vi "SRV_Start Sensors_Build Sensors Commands Arrays.vi"(0 "Sensors Config":T3[](array[typedef]) {"Register" format="%.0x"; "I2C Address" format="%.0x"; "Sample Period (ms)" min=10 max=60000 step=1; "Digital Mask" format="%.0x"; "Channel" format="%.0x"}, 11 "error in (no error)":errorcluster) -> (2 "Streaming Sensor View Indicator Names":T1[](array[typedef]), 3 "Polled Sensor View Indicator Names":T1[](array[typedef]), 6 "Active Streaming Cfg-Commands":T2[](array[typedef]) {"Calculated Sensors Array"."Parsed Formula"."Y Values" format="%.2f"; "Calculated Sensors Array"."Sensor Config"."Register" format="%.0x"; "Calculated Sensors Array"."Sensor Config"."I2C Address" format="%.0x"; "Calculated Sensors Array"."Sensor Config"."Sample Period (ms)" min=10 max=60000 step=1; "Calculated Sensors Array"."Sensor Config"."Digital Mask" format="%.0x"; "Calculated Sensors Array"."Sensor Config"."Channel" format="%.0x"; "Parsed Formula"."Y Values" format="%.2f"; "Sensor Config"."Register" format="%.0x"; "Sensor Config"."I2C Address" format="%.0x"; "Sensor Config"."Sample Period (ms)" min=10 max=60000 step=1; "Sensor Config"."Digital Mask" format="%.0x"; "Sensor Config"."Channel" format="%.0x"}, 10 "Active Polled Cfg-Commands":T2[](array[typedef]) {"Calculated Sensors Array"."Parsed Formula"."Y Values" format="%.2f"; "Calculated Sensors Array"."Sensor Config"."Register" format="%.0x"; "Calculated Sensors Array"."Sensor Config"."I2C Address" format="%.0x"; "Calculated Sensors Array"."Sensor Config"."Sample Period (ms)" min=10 max=60000 step=1; "Calculated Sensors Array"."Sensor Config"."Digital Mask" format="%.0x"; "Calculated Sensors Array"."Sensor Config"."Channel" format="%.0x"; "Parsed Formula"."Y Values" format="%.2f"; "Sensor Config"."Register" format="%.0x"; "Sensor Config"."I2C Address" format="%.0x"; "Sensor Config"."Sample Period (ms)" min=10 max=60000 step=1; "Sensor Config"."Digital Mask" format="%.0x"; "Sensor Config"."Channel" format="%.0x"}, 15 "error out":errorcluster)   [LabVIEW 2009]
uses:
  SRV_Sensor Config Cluster.ctl
  SRV_Sensor Analog-Digital.ctl
  SRV_Sensor Sampling Mode.ctl
  SRV_Sensor View Config Cluster.ctl
  SRV_Sensors Names.ctl
  SRV_Sensor PicoC Shared Var Type.ctl
  SRV_Sensor Number of Bytes.ctl
  SRV_Sensor Integer Word Type.ctl
  SRV_Sensor Config-Command Cluster.ctl
  SRV_Calculated Sensor Cfg.ctl
panel:
  # "operator"
  # "register1"
  # "register2"
  # "operator"
  # "register1"
  # "register2"
  # "operator"
  # "register1"
  # "register2"
  # "operator"
  # "register1"
  # "register2"
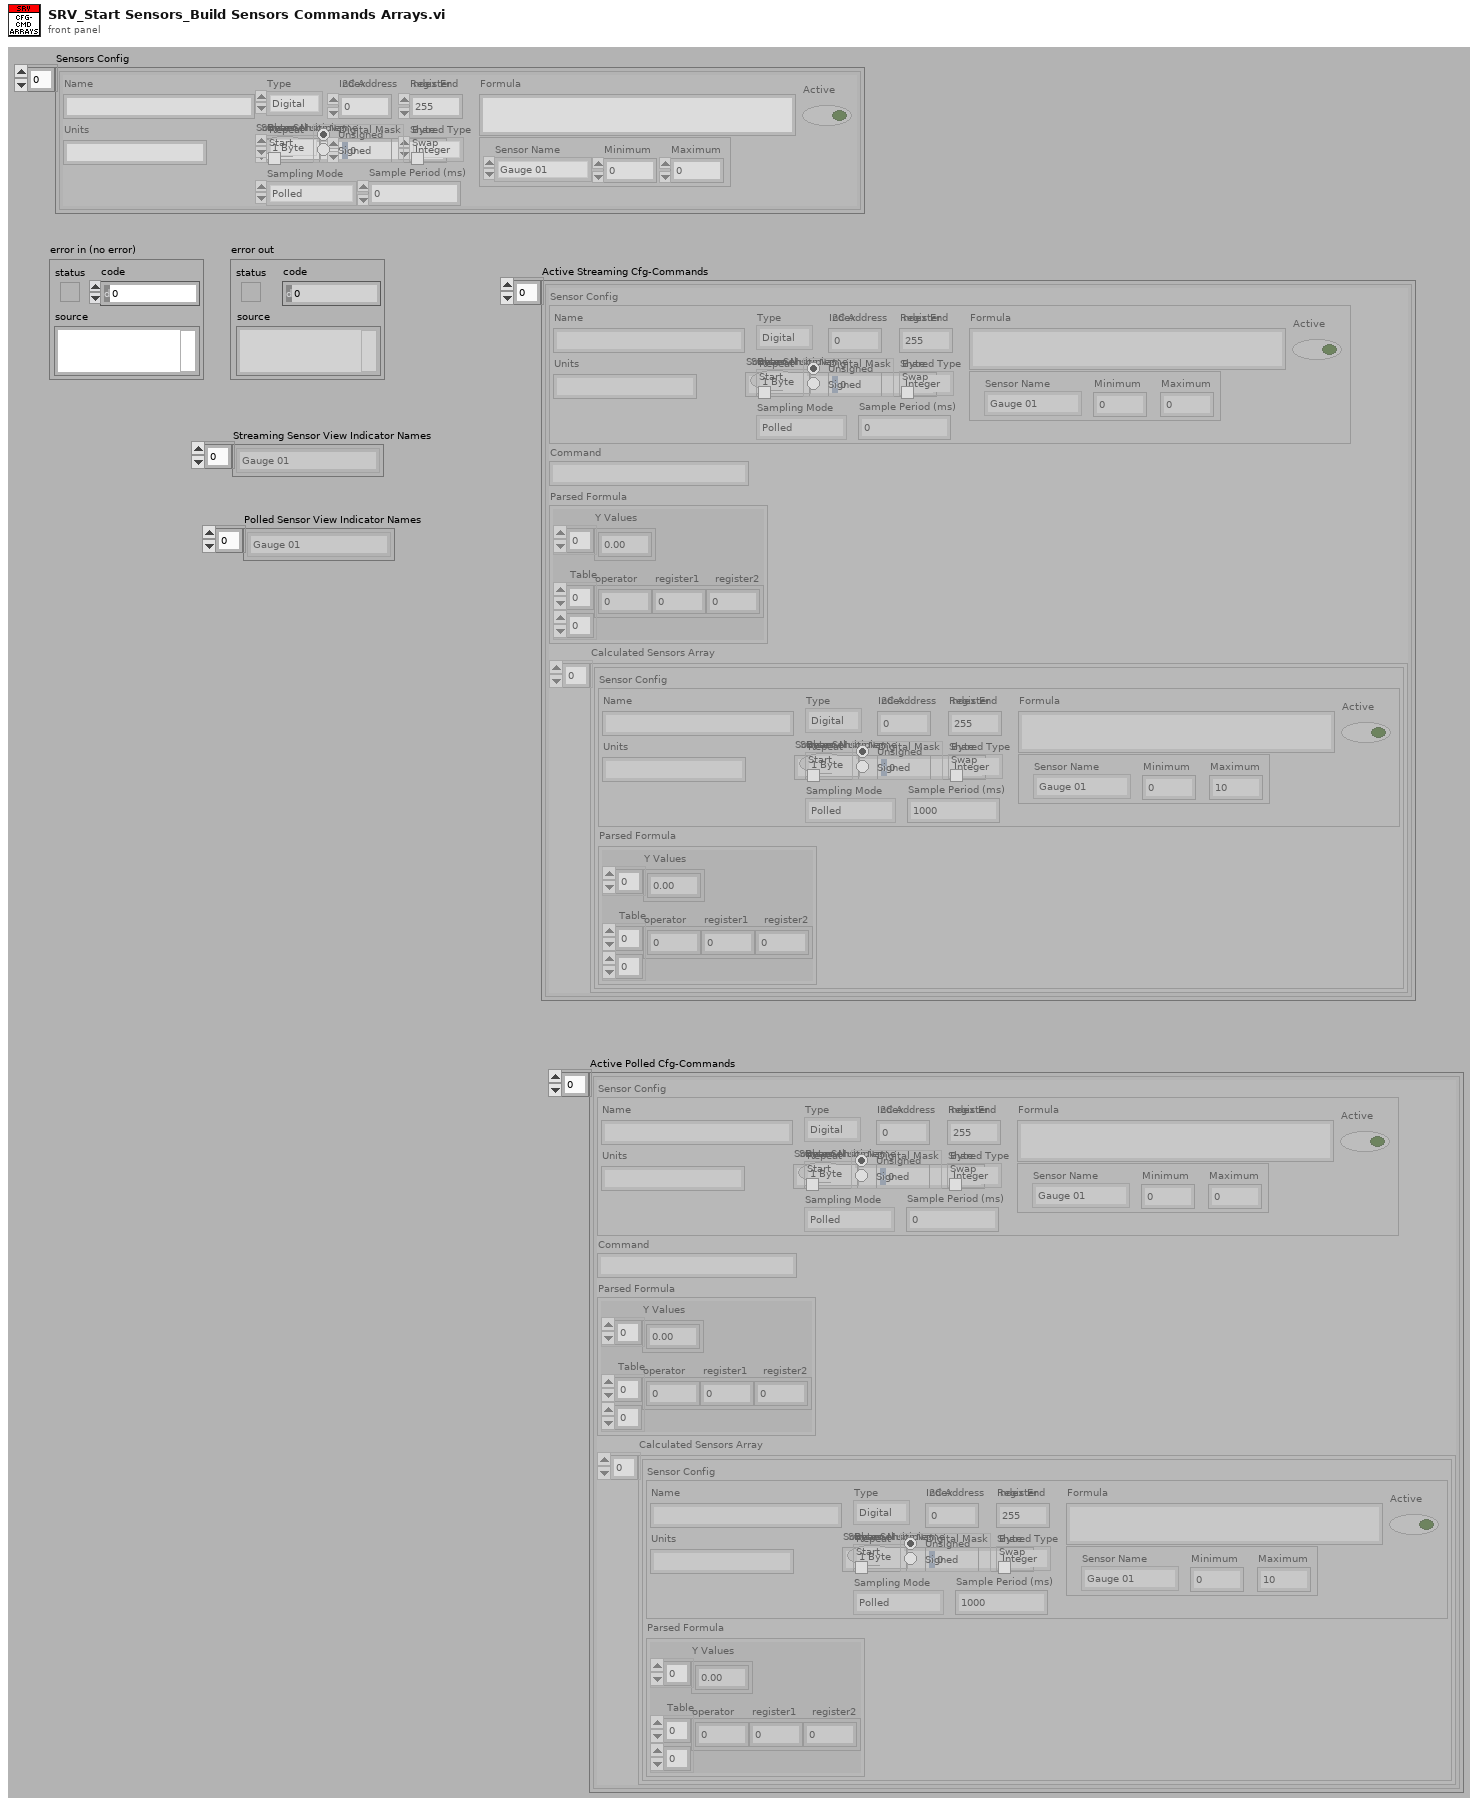
[diagram p1: front panel]
types:
  T1 = typedef "SRV_Sensors Names.ctl" = enum16{"Gauge 01", "Gauge 02", "Gauge 03", "Gauge 04", "Meter 01", "Meter 02", "Meter 03", "Meter 04", "Numeric 01", "Numeric 02", "Numeric 03", "Numeric 04", "Numeric 05", "Numeric 06", "Numeric 07", "Numeric 08", "Boolean 01", "Boolean 02", "Boolean 03", "Boolean 04", "Boolean 05", "Boolean 06", "Boolean 07", "Boolean 08", "Boolean 09", "Boolean 10", "Boolean 11", "Boolean 12", "Boolean 13", "Boolean 14", "Boolean 15", "Boolean 16", "Boolean 17", "Boolean 18", "Boolean 19", "Boolean 20", "Boolean 21", "Boolean 22", "Boolean 23", "Boolean 24", "Boolean 25", "Boolean 26", "Boolean 27", "Boolean 28", "Boolean 29", "Boolean 30", "Boolean 31", "Boolean 32"}
  T2 = typedef "SRV_Sensor Config-Command Cluster.ctl" = cluster{"Sensor Config":T3, "Command":string, "Parsed Formula":cluster{"Table":i32[][], "Y Values":dbl[]}, "Calculated Sensors Array":T10[]}
  T3 = typedef "SRV_Sensor Config Cluster.ctl" = cluster{"Name":string, "A/D":T4, "I2C Address":u8, "Register":u8, "Channel":u8, "Digital Mask":u16, "Units":string, "Sampling Mode":T5, "Sample Period (ms)":u32, "Formula":string, "Sensor View Config":T6, "Active":bool, "PicoC Shared Var Type":T7, "Index":u8, "Stream Multiple?":bool, "Index End":u8, "Bytes":T8, "Source Sensor Name":string, "Repeat Start":bool, "Integer Word Type":T9, "Byte Swap":bool}
  T4 = typedef "SRV_Sensor Analog-Digital.ctl" = enum16{"Digital", "Analog", "PicoC Shared", "Calculated"}
  T5 = typedef "SRV_Sensor Sampling Mode.ctl" = enum16{"Polled", "Streaming"}
  T6 = typedef "SRV_Sensor View Config Cluster.ctl" = cluster{"Sensor Name":T1, "Minimum":dbl, "Maximum":dbl}
  T7 = typedef "SRV_Sensor PicoC Shared Var Type.ctl" = enum16{"String", "Integer", "Float"}
  T8 = typedef "SRV_Sensor Number of Bytes.ctl" = enum16{"1 Byte", "2 Bytes"}
  T9 = typedef "SRV_Sensor Integer Word Type.ctl" = enum32{"Unsigned", "Signed"}
  T10 = typedef "SRV_Calculated Sensor Cfg.ctl" = cluster{"Sensor Config":T3, "Parsed Formula":cluster{"Table":i32[][], "Y Values":dbl[]}}
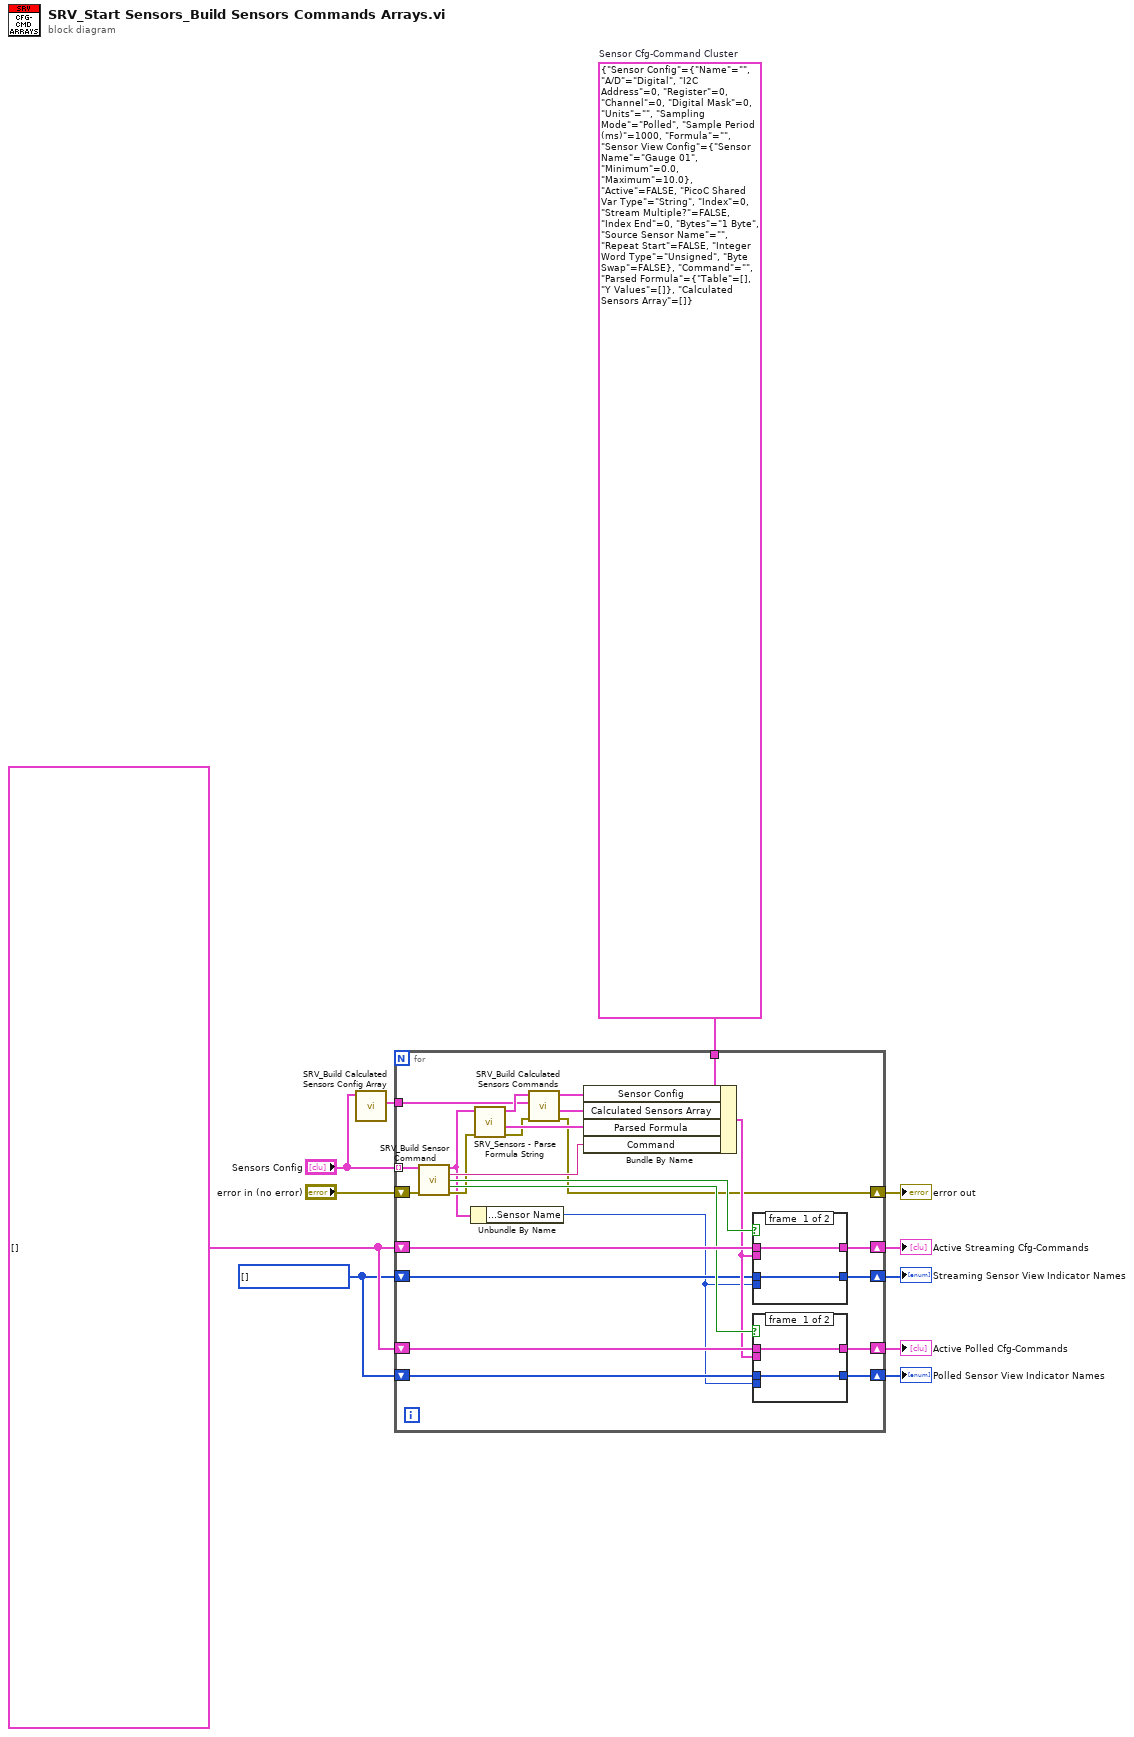
[diagram p0: block diagram]
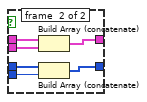
[diagram p2: hidden frame]
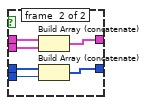
[diagram p3: hidden frame]
diagram:
  w2 = T1[] [] items=["Gauge 01", "Gauge 02", "Gauge 03", "Gauge 04", "Meter 01", "Meter 02", "Meter 03", "Meter 04", "Numeric 01", "Numeric 02", "Numeric 03", "Numeric 04", "Numeric 05", "Numeric 06", "Numeric 07", "Numeric 08", "Boolean 01", "Boolean 02", "Boolean 03", "Boolean 04", "Boolean 05", "Boolean 06", "Boolean 07", "Boolean 08", "Boolean 09", "Boolean 10", "Boolean 11", "Boolean 12", "Boolean 13", "Boolean 14", "Boolean 15", "Boolean 16", "Boolean 17", "Boolean 18", "Boolean 19", "Boolean 20", "Boolean 21", "Boolean 22", "Boolean 23", "Boolean 24", "Boolean 25", "Boolean 26", "Boolean 27", "Boolean 28", "Boolean 29", "Boolean 30", "Boolean 31", "Boolean 32"] ("Sensor View Indicator Names")
  w8 = T2[] []
  w11 = T2 {"Sensor Config"={"Name"="", "A/D"=enum."Digital", "I2C Address"=0, "Register"=0, "Channel"=0, "Digital Mask"=0, "Units"="", "Sampling Mode"=enum."Polled", "Sample Period (ms)"=1000, "Formula"="", "Sensor View Config"={"Sensor Name"=enum."Gauge 01", "Minimum"=0.0, "Maximum"=10.0}, "Active"=FALSE, "PicoC Shared Var Type"=enum."String", "Index"=0, "Stream Multiple?"=FALSE, "Index End"=0, "Bytes"=enum."1 Byte", "Source Sensor Name"="", "Repeat Start"=FALSE, "Integer Word Type"=enum."Unsigned", "Byte Swap"=FALSE}, "Command"="", "Parsed Formula"={"Table"=[], "Y Values"=[]}, "Calculated Sensors Array"=[]}  # Sensor Cfg-Command Cluster
  n1 = call "SRV_Build Calculated Sensors Config Array.vi"("Sensors Config"="Sensors Config") -> ("Calculated Sensors Config"=w4:T3[])  [unwired: 10 in]
  n2 = for {
    tunnel: "Sensors Config" -> [w36] mode=indexing
    shift-right: [w17] -> w10
    shift-left: "error in (no error)" -> [w35]
    tunnel: w11 -> [w34]
    shift-right: [w30] -> w7
    shift-left: w8 -> [w31]
    shift-right: [w29] -> w6
    shift-left: w8 -> [w28]
    shift-right: [w24] -> w3
    shift-left: w2 -> [w25]
    shift-right: [w22] -> w1
    shift-left: w2 -> [w23]
    tunnel: w4 -> [w16]
    n3 = call "SRV_Build Sensor Command.vi"("Sensor Config"=w36, "error in (no error)"=w35) -> ("Sensor Config dup"=w13:T3, "Command"=w33:string, "Active Streaming?"=w32:bool, "Active Polled?"=w27:bool, "error out"=w20:errorcluster)  [unwired: 8 in, 1 out]
    n4 = Unbundle By Name(w13) -> ("Sensor View Config.Sensor Name"=w12:T1)
    n5 = call "SRV_Sensors - Parse Formula String.vi"("error in (no error)"=w20, "Sensor Config"=w13) -> ("error out"=w18:errorcluster, "Parsed Formula"=w21:cluster{"Table":i32[][], "Y Values":dbl[]}, "Sensor Config out"=w19:T3)  [unwired: 7 in]
    n6 = call "SRV_Build Calculated Sensors Commands.vi"("error in (no error)"=w18, "Calculated Sensors Config"=w16, "Sensor Config"=w19) -> ("error out"=w17:errorcluster, "Calculated Sensors Array"=w14:T10[], "Sensor Config dup"=w15:T3)  [unwired: 6 in]
    n7 = Bundle By Name(cluster=w34, "Sensor Config"=w15, "Calculated Sensors Array"=w14, "Parsed Formula"=w21, "Command"=w33) -> (w26:T2)
    n8 = case shown="True" w32 {
      tunnel: w31 -> [w46 w52]
      tunnel: [w46 w50] -> w30
      tunnel: w26 -> [_ w51]
      tunnel: w12 -> [_ w49]
      tunnel: w25 -> [w45 w48]
      tunnel: [w45 w47] -> w24
      frame #0 {
      }
      frame #1 {
        n9 = Build Array (concatenate)(w52, w51) -> (w50:T2[])
        n10 = Build Array (concatenate)(w48, w49) -> (w47:T1[])
      }
    }
    n11 = case shown="True" w27 {
      tunnel: w28 -> [w38 w44]
      tunnel: [w38 w43] -> w29
      tunnel: w26 -> [_ w42]
      tunnel: w12 -> [_ w41]
      tunnel: w23 -> [w37 w40]
      tunnel: [w37 w39] -> w22
      frame #0 {
      }
      frame #1 {
        n12 = Build Array (concatenate)(w44, w42) -> (w43:T2[])
        n13 = Build Array (concatenate)(w40, w41) -> (w39:T1[])
      }
    }
  }
  "error out" <- w10
  "Active Streaming Cfg-Commands" <- w7
  "Active Polled Cfg-Commands" <- w6
  "Streaming Sensor View Indicator Names" <- w3
  "Polled Sensor View Indicator Names" <- w1
